vi "9174_CV_test.vi"() -> ()   [LabVIEW 2015]
uses:
  <vilib>/Utility/sysdir.llb/System Directory Type.ctl
  <vilib>/express/express analysis/Spectral/Block/exnSpectralBlock spectral measurements peak poly.vi
  <vilib>/express/express analysis/Spectral/Block/exnSpectralBlock spectral measurements peak DDT.vi
  <vilib>/express/express analysis/Spectral/XNode/ExpressSpectralMeasurementsBlockNode.xnode
panel:
  out "Save Error out":errorcluster
  out "DAQ Error out":errorcluster
  out "Saving 2":bool
  out "Saving":bool
  in  "Error In":errorcluster
  in  "Stop":bool
  out "tpath":path
  in  "Save Sw":bool
  out "All-Data (Filter)":dynamicdata(graph)
  out "Trigger Val":dynamicdata(graph)
  out "Acc":dynamicdata(graph)
  out "FFT":dynamicdata(graph)
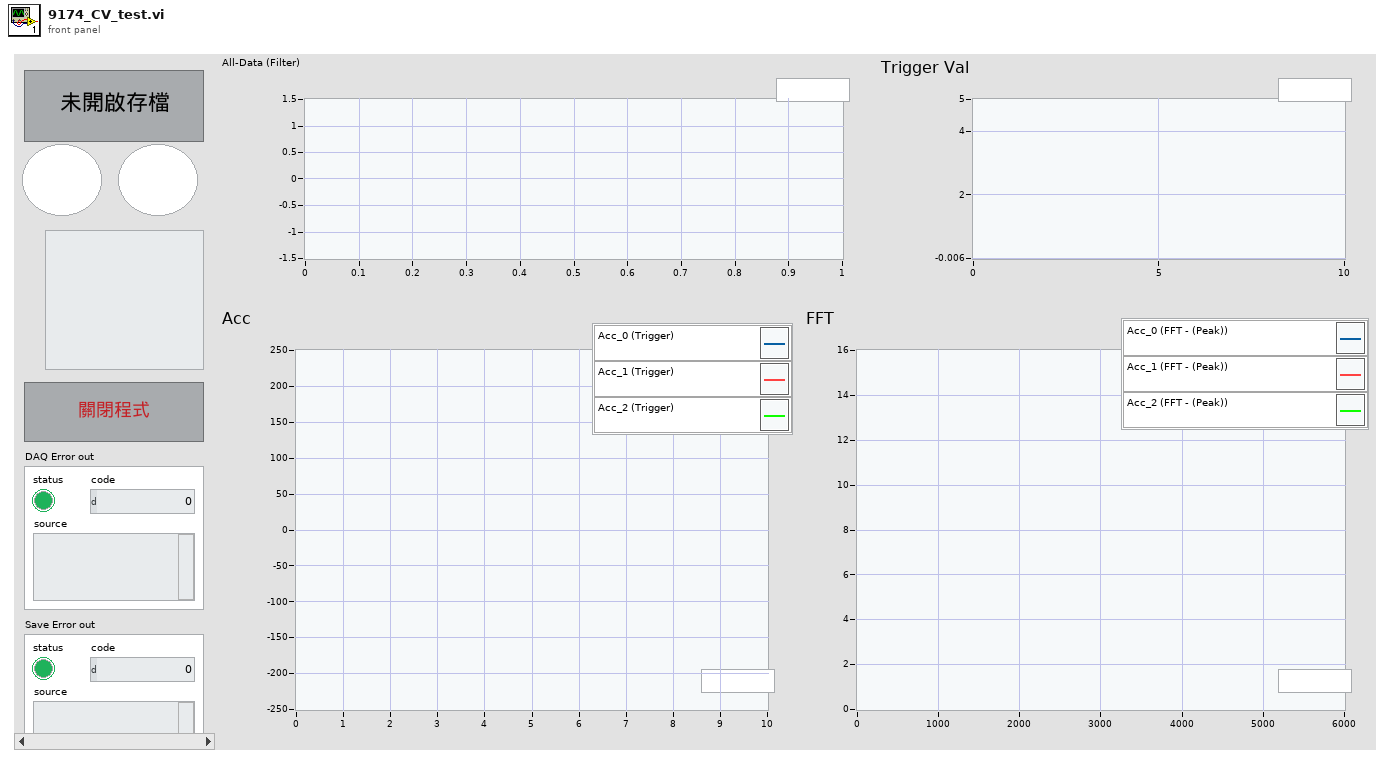
[diagram p1: front panel]
types:
  T1 = typedef "System Directory Type.ctl" = i32
  T2 = cluster{"averaging mode":u16, "weighting mode":u16, "number of averages":u32}
  T3 = cluster{"dB On (F)":bool, "unwrap phase (F)":bool, "convert to degree (F)":bool}
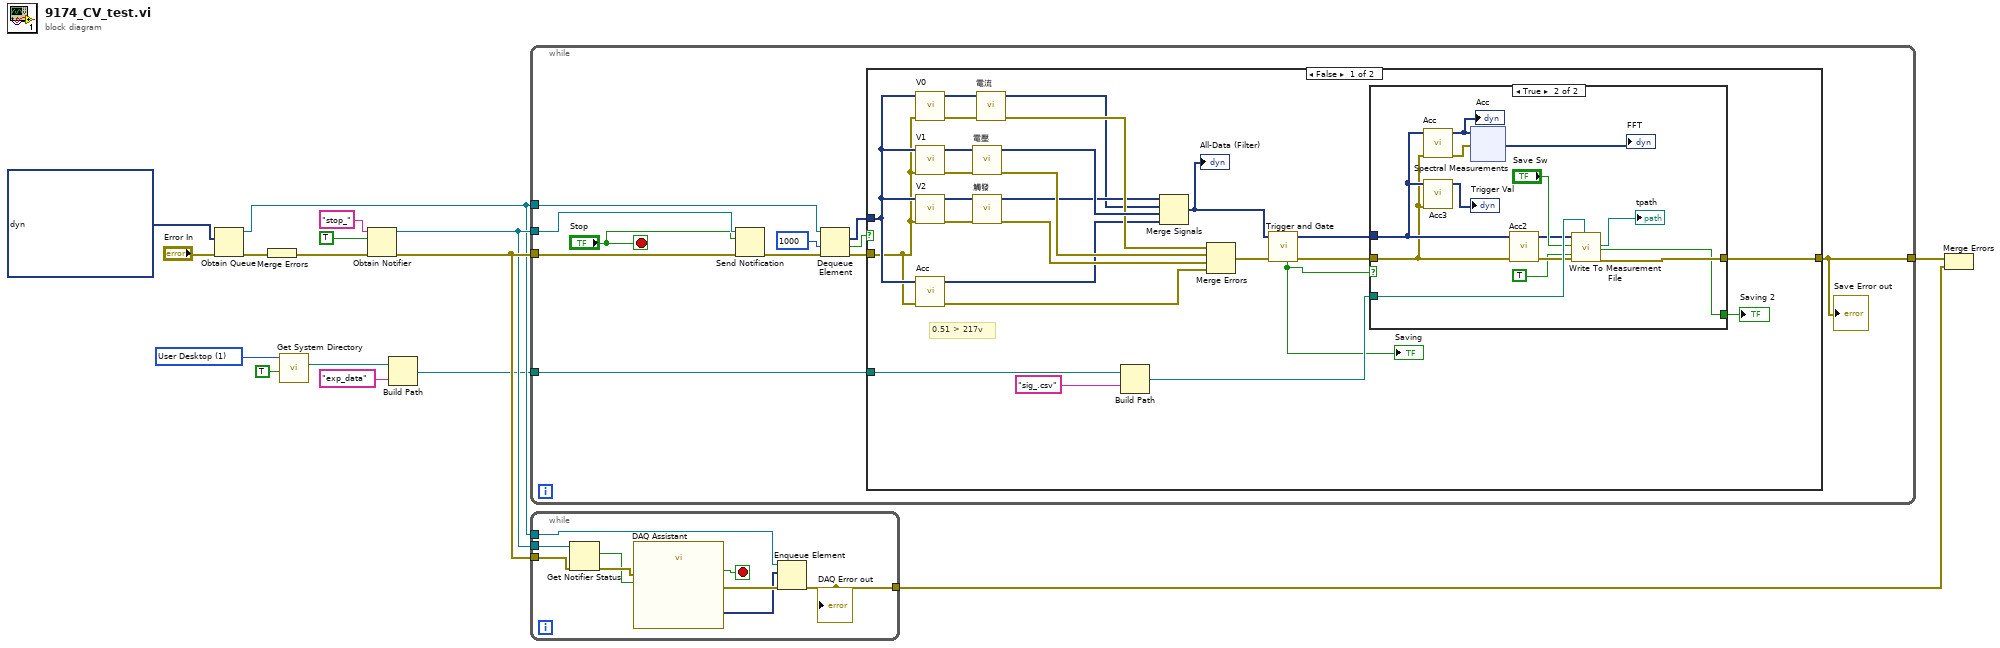
[diagram p0: block diagram]
diagram:
  w2 = T1 1 items=["User Home"=0, "User Desktop"=1, "User Documents"=2, "User Application Data"=3, "User Preferences"=4, "User Temporary"=5, "Public Documents"=6, "Public Application Data"=7, "Public Preferences"=8, "Public Cache"=13, "System Core Libraries"=9, "System Installed Libraries"=10, "Application Files"=11, "Boot Volume Root"=12] ("system directory type")
  n1 = Obtain Queue(element data type=dynamicdata [] ("data"), error in (no error)="Error In") -> (queue out=w6:refnum<queue>, error out=w16:errorcluster)  [unwired: 3 in, 1 out]
  n2 = Merge Errors(w16) -> (w14:errorcluster)
  n3 = call <vilib>:"Get System Directory.vi"("create directory if not found? (F)"=TRUE, "system directory type"=w2) -> ("system directory"=w4:path)  [unwired: 9 in]
  n4 = Obtain Notifier(name (unnamed)="stop_", notification data type=TRUE, error in (no error)=w14) -> (notifier out=w10:refnum<notifier>, error out=w11:errorcluster)  [unwired: 1 in, 1 out]
  n5 = Build Path(base path=w4, name or relative path="exp_data") -> (appended path=w1:path)
  n6 = while {
    tunnel: w11 -> [w27]
    tunnel: w10 -> [w26]
    tunnel: [w17] -> w7
    tunnel: w6 -> [w24]
    tunnel: w1 -> [w18]
    stop <- "Stop" stop-if-true
    n7 = Send Notification(notification="Stop", notifier=w26, error in (no error)=w27) -> (error out=w25:errorcluster)  [unwired: 1 out]
    n8 = Dequeue Element(queue=w24, timeout in ms (-1)=1000, error in (no error)=w25) -> (element=w21:dynamicdata, timed out?=w22:bool, error out=w20:errorcluster)  [unwired: 1 out]
    n9 = case shown="False" w22 {
      tunnel: w21 -> [w40 _]
      tunnel: [w51 w79] -> w17
      tunnel: w20 -> [w33 w79]
      tunnel: w18 -> [w52 _]
      frame False {
        # "0.51 > 217v"
        n10 = call "V0"("error in (no error)"=w33, "Signals"=w40) -> ("error out"=w43:errorcluster, "Signal Out"=w44:dynamicdata)  [unwired: 8 in]
        n11 = call "V1"("error in (no error)"=w33, "Signals"=w40) -> ("error out"=w48:errorcluster, "Signal Out"=w49:dynamicdata)  [unwired: 8 in]
        n12 = call "V2"("error in (no error)"=w33, "Signals"=w40) -> ("error out"=w46:errorcluster, "Signal Out"=w45:dynamicdata)  [unwired: 8 in]
        n13 = call "Acc"("error in (no error)"=w33, "Signals"=w40) -> ("error out"=w29:errorcluster, "Signal Out"=w30:dynamicdata)  [unwired: 8 in]
        n14 = call "電壓"("error in (no error)"=w48, "Signal"=w49) -> ("error out"=w38:errorcluster, "Filtered Signal"=w47:dynamicdata)  [unwired: 8 in]
        n15 = call "觸發"("error in (no error)"=w46, "Signal"=w45) -> ("error out"=w42:errorcluster, "Filtered Signal"=w32:dynamicdata)  [unwired: 8 in]
        n16 = call "電流"("error in (no error)"=w43, "Signal"=w44) -> ("error out"=w41:errorcluster, "Filtered Signal"=w31:dynamicdata)  [unwired: 8 in]
        n17 = Build Path(base path=w52, name or relative path="sig_.csv" ("time format string (%c)")) -> (appended path=w50:path)
        n18 = Merge Signals(w32, w31, w47, w30) -> (w28:dynamicdata)
        "All-Data (Filter)" <- w28
        n19 = Merge Errors(w41, w38, w42, w29) -> (w36:errorcluster)
        n20 = call "Trigger and Gate"("error in (no error)"=w36, "Signals"=w28) -> ("error out"=w35:errorcluster, "Triggered Signals"=w39:dynamicdata, "Data Available"=w37:bool)  [unwired: 6 in, 1 out]
        "Saving" <- w37
        n21 = case shown="True" w37 {
          tunnel: w35 -> [w54 w56]
          tunnel: [w54 w66] -> w51
          tunnel: w50 -> [_ w68]
          tunnel: w39 -> [_ w57]
          tunnel: [_ w65] -> w34
          frame False {
          }
          frame True {
            n22 = call "Acc"("error in (no error)"=w56, "Signals"=w57) -> ("error out"=w60:errorcluster, "Signal Out"=w58:dynamicdata)  [unwired: 8 in]
            "Acc" <- w58
            n23 = call "Acc3"("error in (no error)"=w56, "Signals"=w57) -> ("Signal Out"=→"Trigger Val":dynamicdata)  [unwired: 8 in, 1 out]
            n24 = xnode ("Spectral Measurements")("Signals"=w58, "error in (no error)"=w60) -> ("FFT - (Peak)"=→"FFT":dynamicdata)  [unwired: 2 out]
            n25 = call "Acc2"("error in (no error)"=w56, "Signals"=w57) -> ("error out"=w63:errorcluster, "Signal Out"=w64:dynamicdata)  [unwired: 8 in]
            n26 = call "Write To Measurement File"("Signals"=w64, "Enable"="Save Sw", "new_file"=TRUE, "error in (no error)"=w63, "Filename"=w68) -> ("Filename Out"=→"tpath":path, "Saving Data"=w65:bool, "error out"=w66:errorcluster)  [unwired: 12 in]
          }
        }
        "Saving 2" <- w34
      }
      frame True {
      }
    }
    "Save Error out" <- w17
  }
  n27 = while {
    tunnel: w6 -> [w87]
    tunnel: w11 -> [w84]
    tunnel: w10 -> [w83]
    tunnel: [w80] -> w8
    stop <- w88 stop-if-true
    n28 = Get Notifier Status(notifier=w83, error in (no error)=w84) -> (current notification=w82:bool, error out=w85:errorcluster)  [unwired: 3 out]
    n29 = call "DAQ Assistant"("error in"=w85, "stop (F)"=w82) -> ("data"=w81:dynamicdata, "stopped"=w88:bool, "error out"=w86:errorcluster)  [unwired: 14 in, 1 out]
    n30 = Enqueue Element(queue=w87, element=w81, error in (no error)=w86) -> (error out=w80:errorcluster)  [unwired: 1 in, 2 out]
    "DAQ Error out" <- w80
  }
  n31 = Merge Errors(w7, w8) -> ()  [unwired: 1 out]
